vi "DSF.UDP.Transfer.Set IP Address.vi"(8 "error in (no error)":errorcluster, 10 "IP Address":string="localhost", 11 "UDP Transfer in":refnum<class "DSF.Plugin.UDP.Configuration.Transfer.lvclass">) -> (0 "error out":errorcluster, 3 "UDP Transfer out":refnum<class "DSF.Plugin.UDP.Configuration.Transfer.lvclass">)   [LabVIEW 2016, in "DSF.Plugin.UDP.Configuration.Transfer.lvclass"]
uses:
  DSF.Plugin.UDP.Configuration.Transfer.lvclass
  DSF.Plugin.UDP.Configuration.Transfer.lvclass/DSF.Plugin.UDP.Configuration.Transfer.ctl
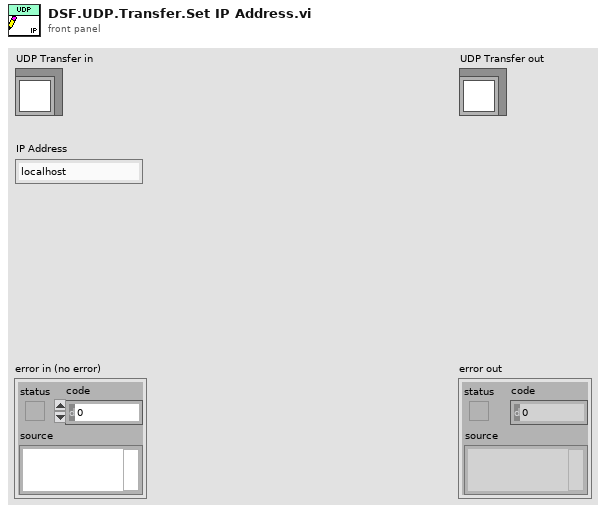
[diagram p1: front panel]
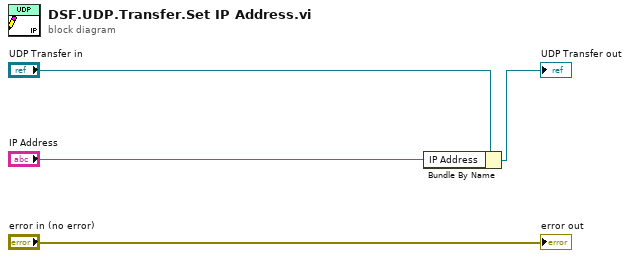
[diagram p0: block diagram]
diagram:
  n1 = Bundle By Name(cluster="UDP Transfer in", "IP Address"="IP Address") -> (→"UDP Transfer out":refnum<class "DSF.Plugin.UDP.Configuration.Transfer.lvclass">)
  "error out" <- "error in (no error)"
